vi "crio_FPGA_Antagonist_DMA.vi"() -> ()   [LabVIEW 2019]
uses:
  <vilib>/rvi/Analysis/control/PID/Typedef/niFpgaPID_PIGains.ctl
  <vilib>/rvi/Analysis/control/PID/Typedef/niFpgaPID_ManualControl.ctl
  hx711/Data.ctl
  hx711/State.ctl
  <vilib>/rvi/Analysis/control/PID/Typedef/niFpgaPID_OutputRange.ctl
  <vilib>/rvi/Emulation/niFpgaSctlEmulationGetInTimedLoop.vi
  <vilib>/rvi/Emulation/niFpgaProcessEmulError.vi
  <vilib>/rvi/eio/common/nirviEmuTemplateMethod_errors.vi
  <vilib>/rvi/Emulation/niFpgaGetClockAttributes.vi
  <vilib>/rvi/Emulation/niFpgaEmulationReportErrorSimple.vi
  <vilib>/rvi/Emulation/niFpgaCriticalErrorInLSC.vi
  <vilib>/rvi/Analysis/control/PID/SubVIs/niFpgaPID_PIWrapper.vi
  <vilib>/rvi/interface/RandomDataEmulation/niFpgaRandomDataHandleErrors.vi
  <vilib>/eio/EIOMethodNode/EIOMethodNode.xnode
  <vilib>/eio/EIONode/EIONode.xnode
  <vilib>/rvi/DataTransferAndStorage/Container/XNode/niFpgaContainer.xnode
  <vilib>/rvi/interface/RandomDataEmulation/nirviRandomDataFpgaReadWriteTemplate.vi
panel:
  out "Data array":i32[](array[numeric])
  in  "PowerDown?":bool
  out "Data":i32
  in  "Gain/ChannelSelect":T1(ring)=enum."Channel A/Gain 64"
  in  "Initial Position":i16=1
  out "Platform Position":i16=20000
  in  "Stepper Direction":bool
  in  "Stepper Enable":bool
  in  "Position Control: Desired Positoin":i16=100
  in  "Manual Operation":bool
  out "Controller Enable":bool
  out "Controller Direction":bool
  in  "mSec to initialize a small push away from limit switch":u32=1 caption="mSec when hit limit"
  in  "mSec when hit limit":u32=100 caption="mSec to pause when hit limit"
  in  "Rail soft limit":i16=10000
  out "Limit Switch":bool
  in  "Half Peirod (pulse 40MHz)":u32=10000 caption="Count(Tick) [Interval between step]"
  out "VCA ControllerPWM Output":sgl
  in  "manual control":T2 {"manual input (0)" scale=-1.0..1.0}
  in  "VCA Position Setpoint":i32
  in  "gains":T3 {"proportional gain" step=0.125}
  in  "Loop Timer DAQ 2":u32=1 caption="Loop Time(uSec)"
  in  "VCA Position Reset":bool
  out "Position (Counts) VCA":i64
  out "B VCA":bool
  out "A VCA":bool
  out "B' VCA":bool
  out "A' VCA":bool
  in  "Velocity Interval (uSec)":u32=1000
  out "Acceleration (Counts/Interval) VCA":i32
  out "Velocity (Counts/Interval) VCA":i32
  in  "DC PWM Period (microsec)":i16=50
  in  "LAC Position":u32(slide)=828 scale=1000.0..2000.0
  in  "Count(uSec)":u32=2000
  in  "stop":bool
  in  "Debug: ConnectorA/DIO15":bool
  in  "Debug: ConnectorA/DIO14":bool
  in  "Encoder Debug":bool
  in  "Loop Timer DAQ":u32=1 caption="Loop Time(uSec)"
  in  "LAC Position Reset":bool
  out "Position (Counts)":i64
  out "B":bool
  out "A":bool
  out "B'":bool
  out "A'":bool
  in  "Velocity Interval (uSec)":u32=1000
  out "Acceleration (Counts/Interval)":i32
  out "Velocity (Counts/Interval)":i32
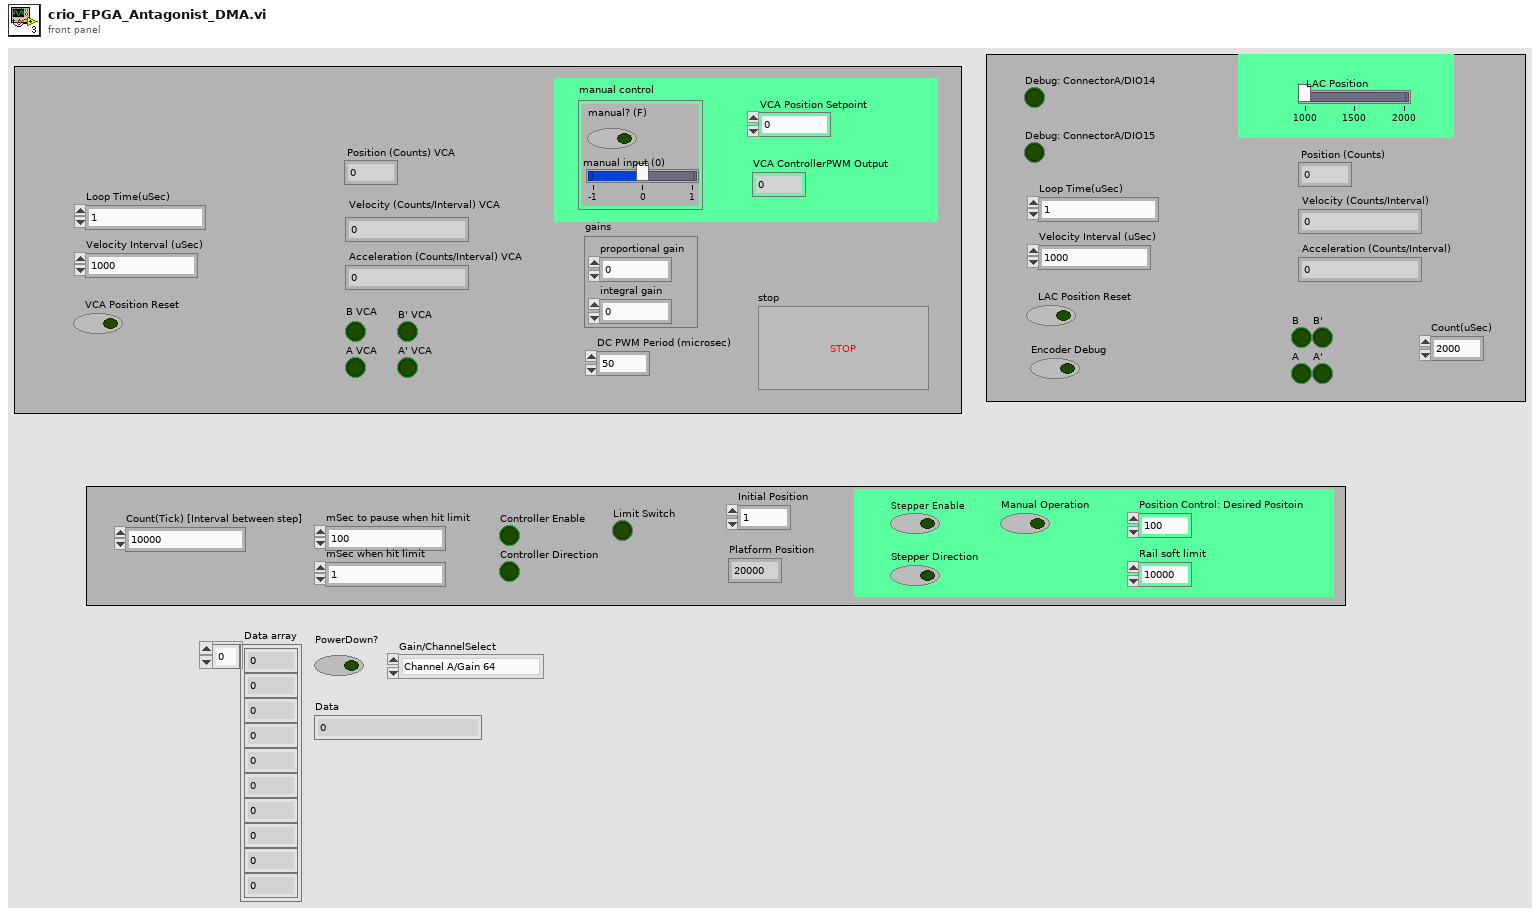
[diagram p1: front panel]
types:
  T1 = enum16{"Channel A/Gain 128", "Channel A/Gain 64", "Channel B/Gain 32"}
  T2 = typedef "niFpgaPID_ManualControl.ctl" = cluster{"manual? (F)":bool, "manual input (0)":sgl}
  T3 = typedef "niFpgaPID_PIGains.ctl" = cluster{"proportional gain":sgl, "integral gain":sgl}
  T4 = typedef "State.ctl" = enum16{"PowerUp", "PowerDown", "Gain/ChannelSelect", "ReadData", "ClockLow", "ClockHigh", "ConvertData", "RetrievalReady?"}
  T5 = typedef "Data.ctl" = cluster{"DT":bool, "SCK":bool, "2's Data":i32, "PulseCount":u8, "DelayTime":u8, "Data":i32, "PowerDown?":bool, "Gain/ChannelSelect":enum16{"Channel A/Gain 128", "Channel A/Gain 64", "Channel B/Gain 32"}}
  T6 = typedef "niFpgaPID_OutputRange.ctl" = cluster{"output high (Inf)":sgl, "output low (-Inf)":sgl}
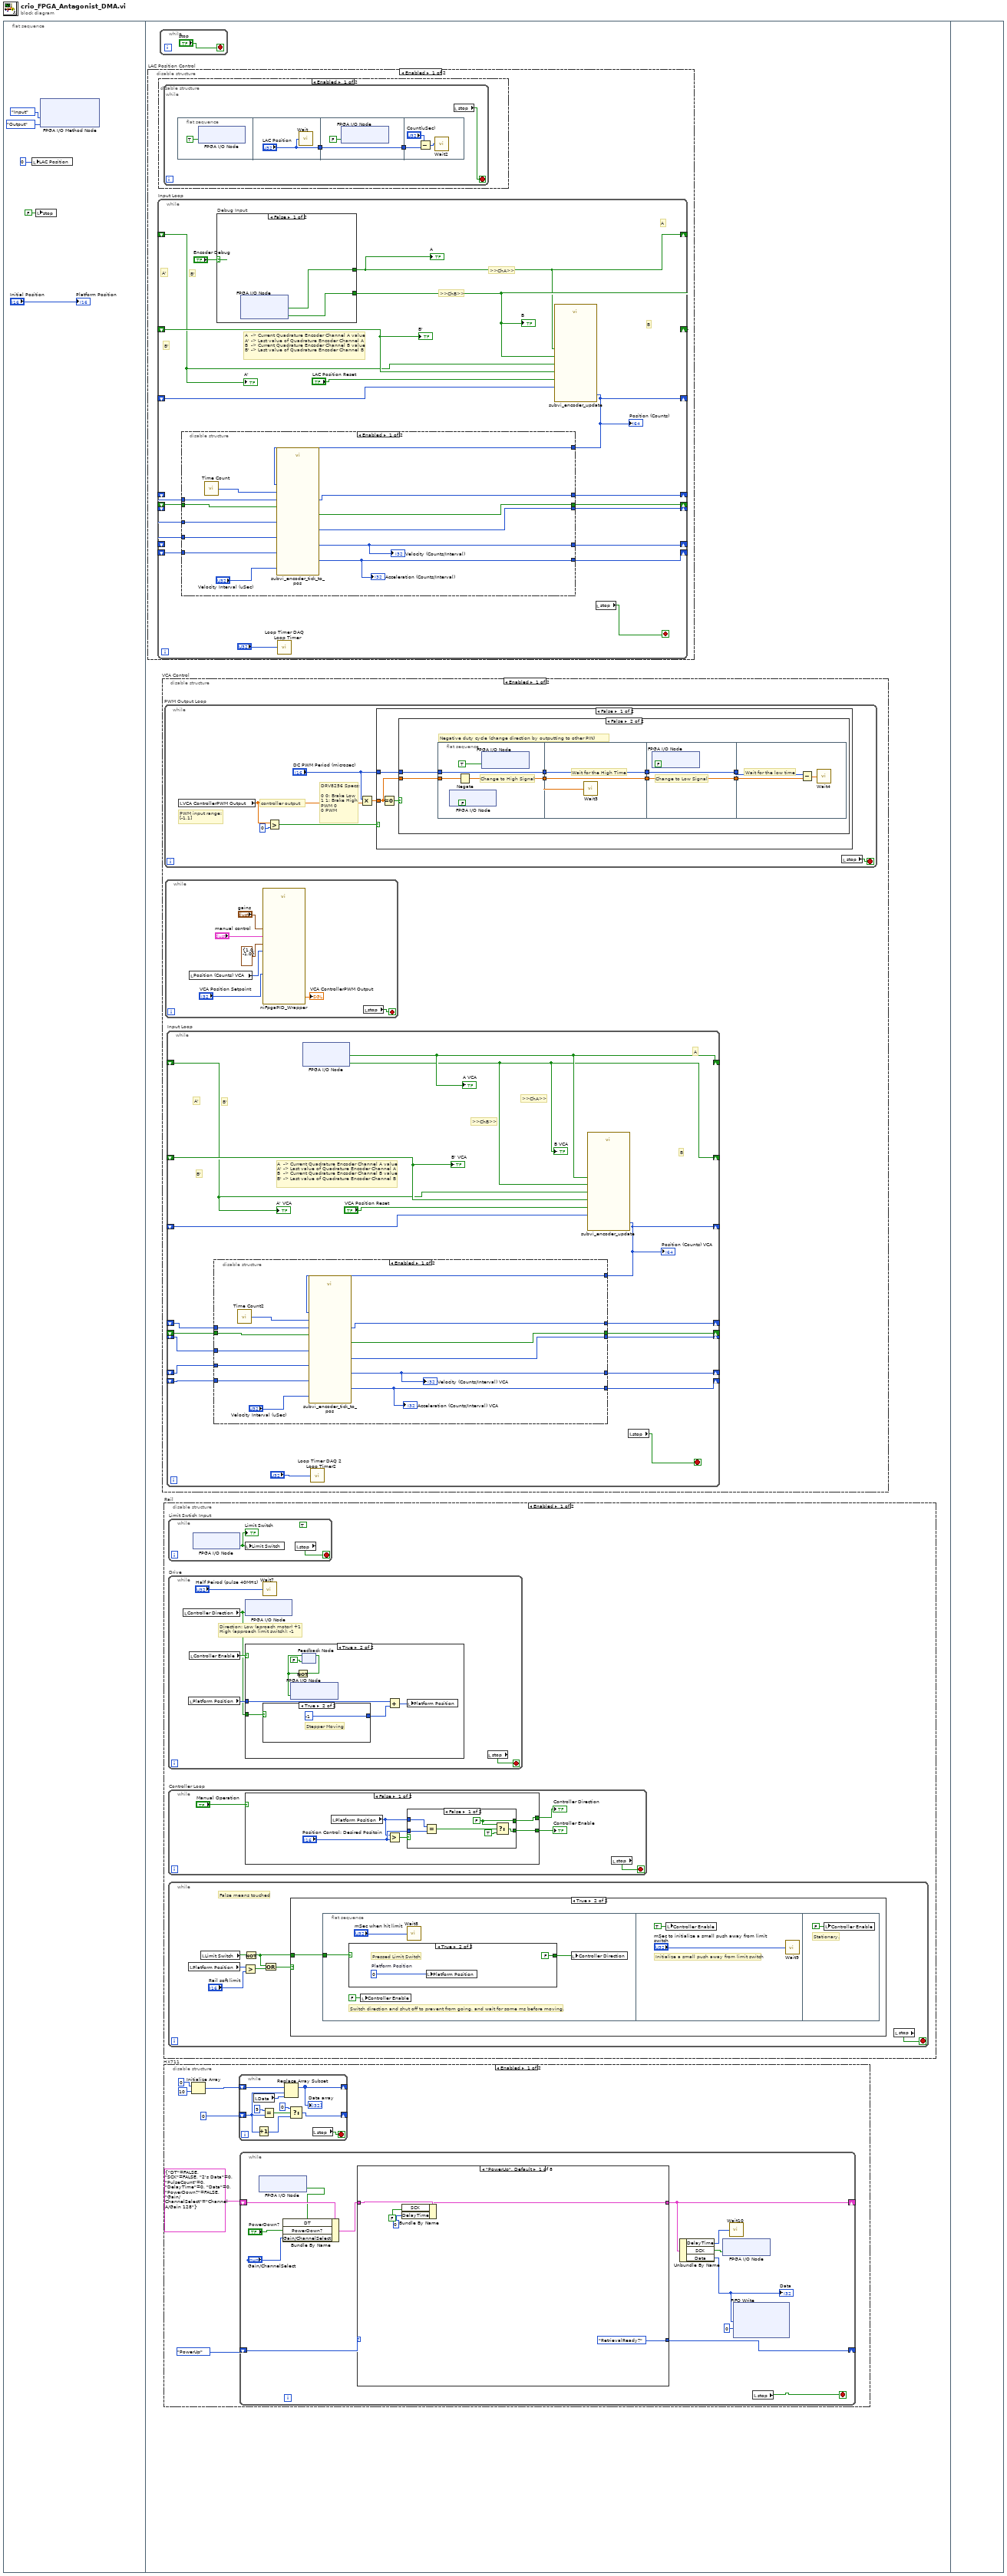
[diagram p0: block diagram]
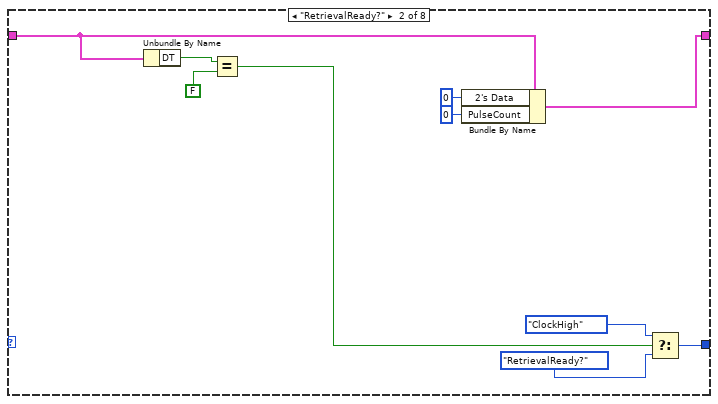
[diagram p2: hidden frame]
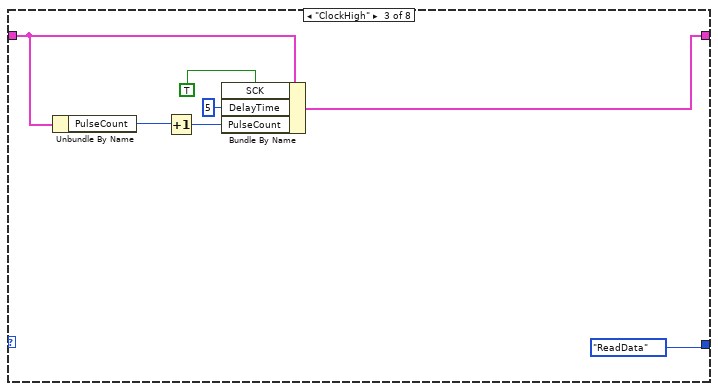
[diagram p3: hidden frame]
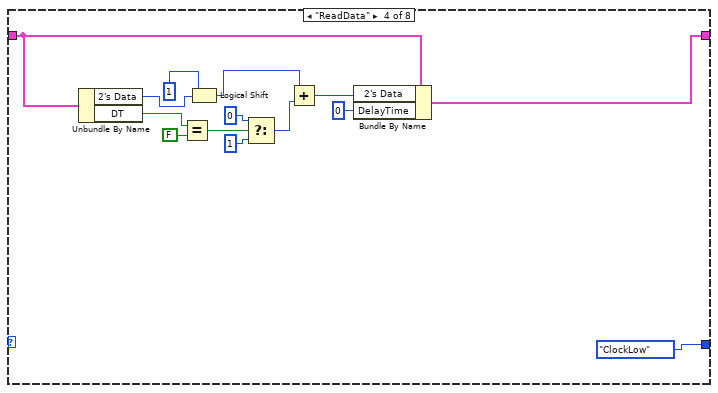
[diagram p4: hidden frame]
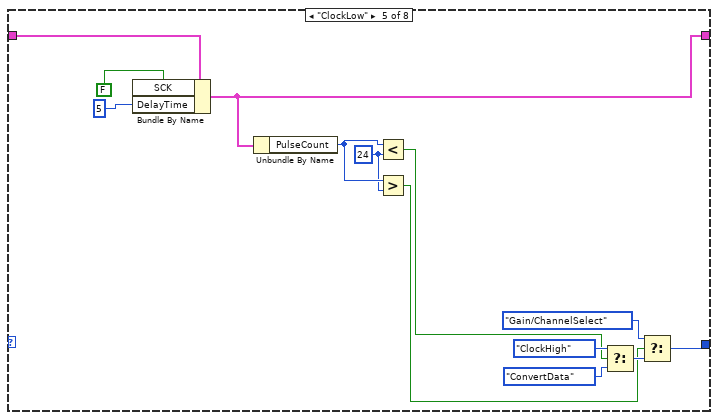
[diagram p5: hidden frame]
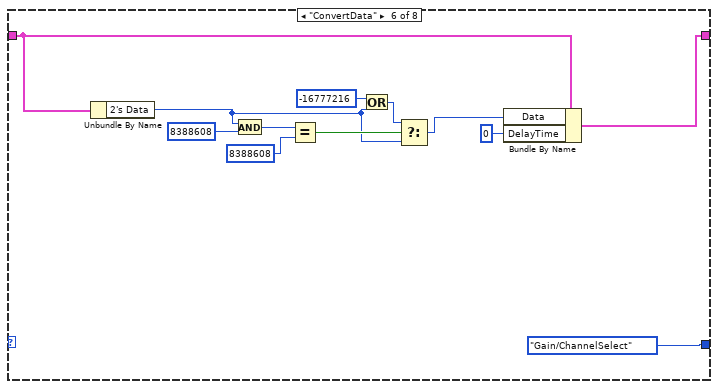
[diagram p6: hidden frame]
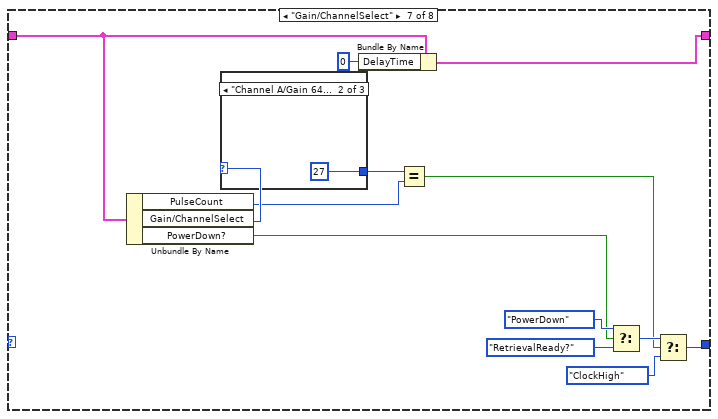
[diagram p7: hidden frame]
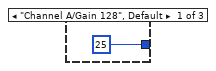
[diagram p8: hidden frame]
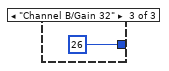
[diagram p9: hidden frame]
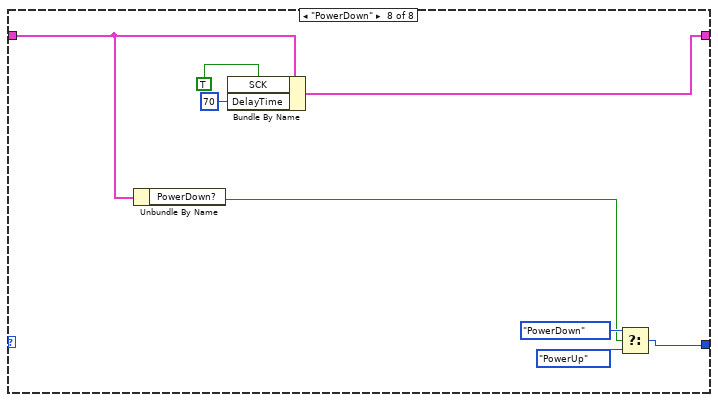
[diagram p10: hidden frame]
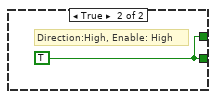
[diagram p12: hidden frame]
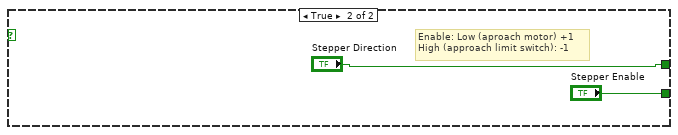
[diagram p13: hidden frame]
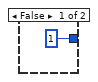
[diagram p15: hidden frame]
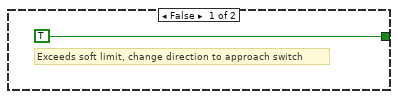
[diagram p17: hidden frame]
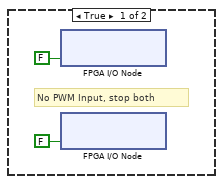
[diagram p20: hidden frame]
diagram:
  n1 = flat-sequence {
    frame #0 {
      n2 = local write "LAC Position"(u32 0 ("Servo wait time")) -> ()
      n3 = local write "stop"(FALSE ("stop")) -> ()
      n4 = xnode "FPGA I/O Method Node"("DIO 7:4"=enum8{"No Change", "Input", "Output"}."Input", "DIO 3:0"=enum8{"No Change", "Input", "Output"}."Output") -> ()  [unwired: 1 in, 1 out]
      "Platform Position" <- "Initial Position"
    }
    frame #1 {
      n5 = disable-structure "LAC Position Control" shown="Enabled" {
        frame Enabled {
          n6 = while "Input Loop" {
            shift-right: [w287] -> _
            shift-left: _ -> [w290]
            shift-right: [w286] -> _
            shift-left: _ -> [w289]
            shift-right: [w282] -> _
            shift-left: _ -> [w288]
            shift-right: [w275] -> _
            shift-left: _ -> [w285]
            shift-right: [w276] -> _
            shift-left: _ -> [w284]
            shift-right: [w283] -> _
            shift-left: _ -> [w281]
            shift-right: [w280] -> _
            shift-left: _ -> [w279]
            shift-right: [w278] -> _
            shift-left: _ -> [w277]
            stop <- w274 stop-if-true
            # "B'"
            # ">>ChB>>"
            # ">>ChA>>"
            # "A'"
            # "A  -> Current Quadrature Encoder Channel A value\nA' -> Last value of Quadrature Encoder Channel A\nB  -> Current Quadrature Encoder Channel B value\nB' -> Last value of Quadrature Encoder Channel B"
            # "B'"
            # "B"
            # "A"
            n7 = case "Debug Input" shown="False" "Encoder Debug" {
              tunnel: [w308 "Debug: ConnectorA/DIO15"] -> w286
              tunnel: [w307 "Debug: ConnectorA/DIO14"] -> w287
              frame False {
                n8 = xnode "FPGA I/O Node"() -> ("Mod1/DIO6"=w308:bool, "Mod1/DIO7"=w307:bool)  [unwired: 2 in, 2 out]
              }
              frame True {
              }
            }
            "B" <- w287
            "A" <- w286
            n9 = call "Loop Timer"("Count(uSec)"="Loop Timer DAQ") -> ()  [unwired: 1 out]
            n10 = call "subvi_encoder_update.vi"("Position Reset"="LAC Position Reset", "Tick'"=w288, "A"=w286, "B'"=w290, "A'"=w289, "B"=w287) -> ("Tick"=w282:i32)  [unwired: 5 in]
            "Position (Counts)" <- w282
            n11 = disable-structure shown="Enabled" {
              disable-tunnel: w285 -> [w305 _]
              disable-tunnel: w284 -> [w304 _]
              disable-tunnel: [w303 _] -> w283
              disable-tunnel: w282 -> [w302 _]
              disable-tunnel: w281 -> [w301 _]
              disable-tunnel: [w300 _] -> w280
              disable-tunnel: w279 -> [w299 _]
              disable-tunnel: [w298 _] -> w278
              disable-tunnel: w277 -> [w297 _]
              disable-tunnel: [w295 _] -> w276
              disable-tunnel: [w294 _] -> w275
              frame Enabled {
                n12 = call "Time Count"() -> ("Tick Count(uSec)"=w296:u32)
                n13 = call "subvi_encoder_tick_to_pos.vi"("Velocity Interval (uSec)"="Velocity Interval (uSec)", "Raw Tick"=w302, "Waited?'"=w299, "Tick Count(uSec)'"=w297, "p'"=w301, "Time Count"=w296, "a'"=w304, "v'"=w305) -> ("Waited?"=w300:bool, "Tick Count(uSec)"=w298:u32, "p"=w303:i32, "a"=w295:i32, "v"=w294:i32)  [unwired: 3 in]
                "Acceleration (Counts/Interval)" <- w295
                "Velocity (Counts/Interval)" <- w294
              }
              frame Disabled {
              }
            }
            n14 = local read "stop"() -> (w274:bool)
            "B'" <- w290
            "A'" <- w289
          }
          n15 = disable-structure shown="Enabled" {
            frame Enabled {
              n16 = while {
                stop <- w264 stop-if-true
                n17 = flat-sequence {
                  tunnel: ["LAC Position"] -> w265
                  tunnel: [w269] -> w266
                  tunnel: w265 -> [w269]
                  tunnel: w266 -> [w273]
                  frame #0 {
                    n18 = xnode "FPGA I/O Node"("Mod8/DIO5"=TRUE) -> ()  [unwired: 1 in, 1 out]
                  }
                  frame #1 {
                    n19 = call "Wait"("Count(uSec)"="LAC Position") -> ()  [unwired: 1 out]
                  }
                  frame #2 {
                    n20 = xnode "FPGA I/O Node"("Mod8/DIO5"=FALSE) -> ()  [unwired: 1 in, 1 out]
                  }
                  frame #3 {
                    n21 = Subtract(x="Count(uSec)", y=w273) -> (x-y=w272:u32)
                    n22 = call "Wait2"("Count(uSec)"=w272) -> ()  [unwired: 1 out]
                  }
                }
                n23 = local read "stop"() -> (w264:bool)
              }
            }
            frame Disabled {
            }
          }
        }
        frame Disabled {
        }
      }
      n24 = while {
        stop <- "stop" stop-if-true
      }
      n25 = disable-structure "VCA Control" shown="Enabled" {
        frame Enabled {
          n26 = while "PWM Output Loop" {
            stop <- w212 stop-if-true
            # "PWM input range:\n[-1,1]"
            # "DRV8256 Specs:\n\n0 0: Brake Low\n1 1: Brake High\nPWM 0\n0 PWM"
            # "controller output"
            n27 = local read "VCA ControllerPWM Output"() -> (w213:sgl)
            n28 = Greater?(x=w213, y=i16 0) -> (0:w216:bool)
            n29 = Multiply(x="DC PWM Period (microsec)", y=w213) -> (x*y=w215:sgl)
            n30 = case shown="False" w216 {
              tunnel: w215 -> [w220 w251]
              tunnel: "DC PWM Period (microsec)" -> [w218 w250]
              frame False {
                n31 = Equal To 0?(x=w220) -> (x = 0?=w219:bool)
                n32 = case shown="False" w219 {
                  tunnel: w220 -> [_ w230]
                  tunnel: w218 -> [_ w223]
                  frame True {
                    # "No PWM Input, stop both"
                    n33 = xnode "FPGA I/O Node"("Mod1/DIO1"=FALSE) -> ()  [unwired: 1 in, 1 out]
                    n34 = xnode "FPGA I/O Node"("Mod1/DIO0"=FALSE) -> ()  [unwired: 1 in, 1 out]
                  }
                  frame False {
                    # "Negative duty cycle (change direction by outputting to other PIN)"
                    n35 = flat-sequence {
                      tunnel: w230 -> [w233]
                      tunnel: [w232] -> w229
                      tunnel: [w231] -> w224
                      tunnel: w223 -> [w231]
                      tunnel: w229 -> [w237]
                      tunnel: [w237] -> w228
                      tunnel: [w236] -> w225
                      tunnel: w224 -> [w236]
                      tunnel: w228 -> [w239]
                      tunnel: [w239] -> w227
                      tunnel: [w238] -> w226
                      tunnel: w225 -> [w238]
                      tunnel: w227 -> [w243]
                      tunnel: w226 -> [w242]
                      frame #0 {
                        # "Change to High Signal"
                        n36 = xnode "FPGA I/O Node"("Mod1/DIO0"=FALSE) -> ()  [unwired: 1 in, 1 out]
                        n37 = Negate(x=w233) -> (-x=w232:sgl)
                        n38 = xnode "FPGA I/O Node"("Mod1/DIO1"=TRUE) -> ()  [unwired: 1 in, 1 out]
                      }
                      frame #1 {
                        # "Wait for the High Time"
                        n39 = call "Wait3"("Count(uSec)"=w237) -> ()  [unwired: 1 out]
                      }
                      frame #2 {
                        # "Change to Low Signal"
                        n40 = xnode "FPGA I/O Node"("Mod1/DIO1"=FALSE) -> ()  [unwired: 1 in, 1 out]
                      }
                      frame #3 {
                        # "Wait for the low time"
                        n41 = Subtract(x=w242, y=w243) -> (x-y=w241:sgl)
                        n42 = call "Wait4"("Count(uSec)"=w241) -> ()  [unwired: 1 out]
                      }
                    }
                  }
                }
              }
              frame True {
                n43 = flat-sequence {
                  tunnel: w251 -> [w252]
                  tunnel: w250 -> [w253]
                  tunnel: [w253] -> w247
                  tunnel: [w252] -> w246
                  tunnel: [w257] -> w248
                  tunnel: w247 -> [w257]
                  tunnel: w246 -> [w256]
                  tunnel: [w256] -> w245
                  tunnel: [w259] -> w249
                  tunnel: w248 -> [w259]
                  tunnel: w245 -> [w258]
                  tunnel: [w258] -> w244
                  tunnel: w249 -> [w263]
                  tunnel: w244 -> [w261]
                  frame #0 {
                    # "Change to High Signal"
                    n44 = xnode "FPGA I/O Node"("Mod1/DIO1"=FALSE ("ConnectorB/DIO9")) -> ()  [unwired: 1 in, 1 out]
                    n45 = xnode "FPGA I/O Node"("Mod1/DIO0"=TRUE) -> ()  [unwired: 1 in, 1 out]
                  }
                  frame #1 {
                    # "Wait for the high time"
                    n46 = call "Wait5"("Count(uSec)"=w256) -> ()  [unwired: 1 out]
                  }
                  frame #2 {
                    # "Turn off"
                    n47 = xnode "FPGA I/O Node"("Mod1/DIO0"=FALSE) -> ()  [unwired: 1 in, 1 out]
                  }
                  frame #3 {
                    # "Wait for the low time"
                    n48 = Subtract(x=w263, y=w261) -> (x-y=w262:sgl)
                    n49 = call "Wait6"("Count(uSec)"=w262) -> ()  [unwired: 1 out]
                  }
                }
              }
            }
            n50 = local read "stop"() -> (w212:bool)
          }
          n51 = while {
            stop <- w211 stop-if-true
            n52 = local read "Position (Counts) VCA"() -> (w210:i64)
            n53 = call-poly <vilib>:"niFpgaPID_Wrapper.vi"("setpoint"="VCA Position Setpoint", "process variable"=w210, "manual control"="manual control", "gains"="gains", "output range"=T6 {"output high (Inf)"=1.0, "output low (-Inf)"=-1.0}) -> ("output"=→"VCA ControllerPWM Output":sgl)  [unwired: 8 in, 2 out]
            n54 = local read "stop"() -> (w211:bool)
          }
          n55 = while "Input Loop" {
            shift-right: [w173] -> _
            shift-left: _ -> [w189]
            shift-right: [w174] -> _
            shift-left: _ -> [w188]
            shift-right: [w183] -> _
            shift-left: _ -> [w187]
            shift-right: [w176] -> _
            shift-left: _ -> [w186]
            shift-right: [w177] -> _
            shift-left: _ -> [w185]
            shift-right: [w184] -> _
            shift-left: _ -> [w182]
            shift-right: [w181] -> _
            shift-left: _ -> [w180]
            shift-right: [w179] -> _
            shift-left: _ -> [w178]
            stop <- w175 stop-if-true
            # "B'"
            # ">>ChB>>"
            # ">>ChA>>"
            # "A'"
            # "A  -> Current Quadrature Encoder Channel A value\nA' -> Last value of Quadrature Encoder Channel A\nB  -> Current Quadrature Encoder Channel B value\nB' -> Last value of Quadrature Encoder Channel B"
            # "B'"
            # "B"
            # "A"
            n56 = xnode "FPGA I/O Node"() -> ("Mod1/DIO4"=w174:bool, "Mod1/DIO5"=w173:bool)  [unwired: 2 in, 2 out]
            "B VCA" <- w173
            "A VCA" <- w174
            n57 = call "Loop Timer2"("Count(uSec)"="Loop Timer DAQ 2") -> ()  [unwired: 1 out]
            n58 = call "subvi_encoder_update.vi"("Position Reset"="VCA Position Reset", "Tick'"=w187, "A"=w174, "B'"=w189, "A'"=w188, "B"=w173) -> ("Tick"=w183:i32)  [unwired: 5 in]
            "Position (Counts) VCA" <- w183
            n59 = disable-structure shown="Enabled" {
              disable-tunnel: w186 -> [w203 _]
              disable-tunnel: w185 -> [w202 _]
              disable-tunnel: [w201 _] -> w184
              disable-tunnel: w183 -> [w200 _]
              disable-tunnel: w182 -> [w199 _]
              disable-tunnel: [w198 _] -> w181
              disable-tunnel: w180 -> [w197 _]
              disable-tunnel: [w196 _] -> w179
              disable-tunnel: w178 -> [w195 _]
              disable-tunnel: [w193 _] -> w177
              disable-tunnel: [w192 _] -> w176
              frame Enabled {
                n60 = call "Time Count2"() -> ("Tick Count(uSec)"=w194:u32)
                n61 = call "subvi_encoder_tick_to_pos.vi"("Velocity Interval (uSec)"="Velocity Interval (uSec)", "Raw Tick"=w200, "Waited?'"=w197, "Tick Count(uSec)'"=w195, "p'"=w199, "Time Count"=w194, "a'"=w202, "v'"=w203) -> ("Waited?"=w198:bool, "Tick Count(uSec)"=w196:u32, "p"=w201:i32, "a"=w193:i32, "v"=w192:i32)  [unwired: 3 in]
                "Acceleration (Counts/Interval) VCA" <- w193
                "Velocity (Counts/Interval) VCA" <- w192
              }
              frame Disabled {
              }
            }
            n62 = local read "stop"() -> (w175:bool)
            "B' VCA" <- w189
            "A' VCA" <- w188
          }
        }
        frame Disabled {
        }
      }
      n63 = disable-structure "Rail" shown="Enabled" {
        frame Enabled {
          n64 = while "Limit Swtich Input" {
            stop <- w171 stop-if-true
            (unwired) TRUE ("Mod8/DIO2")
            n65 = xnode "FPGA I/O Node"() -> ("Mod8/DIO2"=w172:bool)  [unwired: 1 in, 1 out]
            "Limit Switch" <- w172
            n66 = local write "Limit Switch"(w172) -> ()
            n67 = local read "stop"() -> (w171:bool)
          }
          n68 = while "Drive" {
            stop <- w139 stop-if-true
            # "Direction: Low (aproach motor) +1\nHigh (approach limit switch): -1"
            n69 = local read "Controller Direction"() -> (w140:bool)
            n70 = local read "Platform Position"() -> (w142:i16)
            n71 = local read "Controller Enable"() -> (w141:bool)
            n72 = xnode "FPGA I/O Node"("Mod8/DIO4"=w140) -> ()  [unwired: 1 in, 1 out]
            n73 = case shown="True" w141 {
              tunnel: w140 -> [_ w147]
              tunnel: w142 -> [_ w144]
              frame False {
              }
              frame True {
                n74 = case shown="True" w147 {
                  tunnel: [i16 1 i16 -1] -> w146
                  frame False {
                  }
                  frame True {
                    # "Stepper Moving"
                  }
                }
                n75 = feedback #1(FALSE ("Connector0/DIO0")) -> (w148:bool)
                n76 = xnode "FPGA I/O Node"("Mod8/DIO3"=w148) -> ()  [unwired: 1 in, 1 out]
                n77 = Not(x=w148) -> (.not. x?=w149:bool)
                n78 = feedback-in #1(w149) -> ()
                n79 = Add(x=w144, y=w146) -> (x+y=w145:i16)
                n80 = local write "Platform Position"(w145) -> ()
              }
            }
            n81 = call "Wait7"("Count(Ticks)"="Half Peirod (pulse 40MHz)") -> ()  [unwired: 1 out]
            n82 = local read "stop"() -> (w139:bool)
          }
          n83 = while "Controller Loop" {
            stop <- w124 stop-if-true
            n84 = case shown="False" "Manual Operation" {
              tunnel: [w128 "Stepper Enable"] -> w122
              tunnel: [w127 "Stepper Direction"] -> w121
              frame False {
                n85 = local read "Platform Position"() -> (w125:i16)
                n86 = Greater?(x=w125, y="Position Control: Desired Positoin") -> (0:w129:bool)
                n87 = case shown="False" w129 {
                  tunnel: [w132 w136] -> w128
                  tunnel: [w130 w136] -> w127
                  tunnel: "Position Control: Desired Positoin" -> [w135 _]
                  tunnel: w125 -> [w134 _]
                  frame False {
                    w130 = FALSE
                    n88 = Equal?(x=w134, y=w135) -> (x = y?=w133:bool)
                    n89 = Select(t=w130, s=w133, f=TRUE) -> (s? t:f=w132:bool)
                  }
                  frame True {
                    w136 = TRUE
                    # "Direction:High, Enable: High"
                  }
                }
              }
              frame True {
                # "Enable: Low (aproach motor) +1\nHigh (approach limit switch): -1"
              }
            }
            "Controller Enable" <- w122
            "Controller Direction" <- w121
            n90 = local read "stop"() -> (w124:bool)
          }
          n91 = while {
            stop <- w159 stop-if-true
            # "False means touched"
            n92 = local read "Platform Position"() -> (w158:i16)
            n93 = local read "Limit Switch"() -> (w154:bool)
            n94 = Greater?(x=w158, y="Rail soft limit") -> (0:w156:bool)
            n95 = Not(x=w154) -> (.not. x?=w153:bool)
            n96 = Or(x=w153, y=w156) -> (x .or. y?=w155:bool)
            n97 = case shown="True" w155 {
              tunnel: w153 -> [_ w160]
              frame False {
                # "Do nothing"
              }
              frame True {
                n98 = flat-sequence {
                  tunnel: w160 -> [w161]
                  frame #0 {
                    # "Switch direction and shut off to prevent from going, and wait for some ms before moving."
                    n99 = case shown="True" w161 {
                      tunnel: [TRUE ("Stepper Direction") FALSE ("Stepper Direction")] -> w162
                      frame False {
                        # "Exceeds soft limit, change direction to approach switch"
                      }
                      frame True {
                        w167 = i16 0  # Platform Position
                        # "Pressed Limit Switch"
                        n100 = local write "Platform Position"(w167) -> ()
                      }
                    }
                    n101 = local write "Controller Enable"(FALSE ("Stepper Direction")) -> ()
                    n102 = call "Wait8"("Count(mSec)"="mSec when hit limit") -> ()  [unwired: 1 out]
                    n103 = local write "Controller Direction"(w162) -> ()
                  }
                  frame #1 {
                    # "Initialize a small push away from limit switch"
                    n104 = local write "Controller Enable"(TRUE ("Stepper Enable")) -> ()
                    n105 = call "Wait9"("Count(mSec)"="mSec to initialize a small push away from limit switch") -> ()  [unwired: 1 out]
                  }
                  frame #2 {
                    # "Stationary."
                    n106 = local write "Controller Enable"(FALSE ("Stepper Enable")) -> ()
                  }
                }
              }
            }
            n107 = local read "stop"() -> (w159:bool)
          }
        }
        frame Disabled {
        }
      }
      n108 = disable-structure "HX711" shown="Enabled" {
        frame Enabled {
          n109 = Initialize Array(0 ("Data"), 10 ("dimension size")) -> (w12:i32[])
          n110 = while {
            shift-right: [w112] -> _
            shift-left: w12 -> [w113]
            shift-right: [w118] -> _
            shift-left: 0 ("index") -> [w114]
            stop <- w111 stop-if-true
            n111 = local read "Data"() -> (w120:i32)
            n112 = Increment(x=w114) -> (x+1=w117:i32)
            n113 = Equal?(x=9, y=w114) -> (x = y?=w115:bool)
            n114 = Replace Array Subset(array=w113, new element=w120, index=w114) -> (w112:i32[])
            "Data array" <- w112
            n115 = Select(t=0 ("index"), s=w115, f=w117) -> (s? t:f=w118:i32)
            n116 = local read "stop"() -> (w111:bool)
          }
          n117 = while {
            shift-right: [w17] -> _
            shift-left: T5 {"DT"=FALSE, "SCK"=FALSE, "2's Data"=0, "PulseCount"=0, "DelayTime"=0, "Data"=0, "PowerDown?"=FALSE, "Gain/ChannelSelect"=enum."Channel A/Gain 128"} ("Data") -> [w22]
            shift-right: [w23] -> _
            shift-left: State."PowerUp" ("State") -> [w25]
            stop <- w15 stop-if-true
            n118 = xnode "FPGA I/O Node"() -> ("Mod8/DIO0"=w20:bool)  [unwired: 1 in, 1 out]
            n119 = Bundle By Name(cluster=w22, "DT"=w20, "PowerDown?"="PowerDown?", "Gain/ChannelSelect"="Gain/ChannelSelect") -> (w21:T5)
            n120 = case shown="\"PowerUp\", Default" w25 {
              tunnel: w21 -> [w30 w34 w43 w48 w74 w79 w89 w104]
              tunnel: [w28 w33 w47 w50 w69 w78 w88 w110] -> w17
              tunnel: [State."RetrievalReady?" ("State") w36 State."ReadData" ("State") State."ClockLow" ("State") w70 State."Gain/ChannelSelect" ("State") w96 w105] -> w23
              frame "PowerUp", Default {
                n121 = Bundle By Name(cluster=w30, "SCK"=FALSE, "DelayTime"=u8 0) -> (w28:T5)
              }
              frame "RetrievalReady?" {
                n122 = Unbundle By Name(w34) -> ("DT"=w40:bool)
                n123 = Equal?(x=w40, y=FALSE) -> (x = y?=w35:bool)
                n124 = Bundle By Name(cluster=w34, "2's Data"=0, "PulseCount"=u8 0) -> (w33:T5)
                n125 = Select(t=State."ClockHigh" ("State"), s=w35, f=State."RetrievalReady?" ("State")) -> (s? t:f=w36:T4)
              }
              frame "ClockHigh" {
                n126 = Unbundle By Name(w43) -> ("PulseCount"=w42:u8)
                n127 = Increment(x=w42) -> (x+1=w41:u8)
                n128 = Bundle By Name(cluster=w43, "SCK"=TRUE, "DelayTime"=u8 5, "PulseCount"=w41) -> (w47:T5)
              }
              frame "ReadData" {
                n129 = Unbundle By Name(w48) -> ("2's Data"=w61:i32, "DT"=w59:bool)
                n130 = Equal?(x=w59, y=FALSE ("SCK")) -> (x = y?=w57:bool)
                n131 = Logical Shift(y=i16 1, x=w61) -> (x << y=w56:i32)
                n132 = Select(t=0 ("DelayTime"), s=w57, f=1 ("DelayTime")) -> (s? t:f=w53:i32)
                n133 = Add(x=w56, y=w53) -> (x+y=w52:i32)
                n134 = Bundle By Name(cluster=w48, "2's Data"=w52, "DelayTime"=u8 0) -> (w50:T5)
              }
              frame "ClockLow" {
                w63 = u8 24 ("y")
                n135 = Bundle By Name(cluster=w74, "SCK"=FALSE, "DelayTime"=u8 5) -> (w69:T5)
                n136 = Unbundle By Name(w69) -> ("PulseCount"=w64:u8)
                n137 = Less?(x=w64, y=w63) -> (x < y?=w66:bool)
                n138 = Greater?(x=w64, y=w63) -> (0:w62:bool)
                n139 = Select(t=State."ClockHigh" ("State"), s=w66, f=State."ConvertData" ("State")) -> (s? t:f=w65:T4)
                n140 = Select(t=State."Gain/ChannelSelect" ("State"), s=w62, f=w65) -> (s? t:f=w70:T4)
              }
              frame "ConvertData" {
                n141 = Unbundle By Name(w79) -> ("2's Data"=w80:i32)
                n142 = And(x=w80, y=8388608) -> (x .and. y?=w85:i32)
                n143 = Equal?(x=w85, y=8388608) -> (x = y?=w83:bool)
                n144 = Or(x=-16777216 ("y"), y=w80) -> (x .or. y?=w81:i32)
                n145 = Select(t=w81, s=w83, f=w80) -> (s? t:f=w76:i32)
                n146 = Bundle By Name(cluster=w79, "Data"=w76, "DelayTime"=u8 0) -> (w78:T5)
              }
              frame "Gain/ChannelSelect" {
                n147 = Unbundle By Name(w89) -> ("PulseCount"=w92:u8, "Gain/ChannelSelect"=w94:T1, "PowerDown?"=w95:bool)
                n148 = case shown="\"Channel A/Gain 64\"" w94 {
                  tunnel: [u8 25 ("PulseCount") u8 27 ("PulseCount") u8 26 ("PulseCount")] -> w93
                  frame "Channel A/Gain 128", Default {
                  }
                  frame "Channel A/Gain 64" {
                  }
                  frame "Channel B/Gain 32" {
                  }
                }
                n149 = Bundle By Name(cluster=w89, "DelayTime"=u8 0) -> (w88:T5)
                n150 = Equal?(x=w93, y=w92) -> (x = y?=w90:bool)
                n151 = Select(t=State."PowerDown" ("State"), s=w95, f=State."RetrievalReady?" ("State")) -> (s? t:f=w91:T4)
                n152 = Select(t=w91, s=w90, f=State."ClockHigh" ("State")) -> (s? t:f=w96:T4)
              }
              frame "PowerDown" {
                n153 = Unbundle By Name(w104) -> ("PowerDown?"=w103:bool)
                n154 = Bundle By Name(cluster=w104, "SCK"=TRUE, "DelayTime"=u8 70) -> (w110:T5)
                n155 = Select(t=State."PowerDown" ("State"), s=w103, f=State."PowerUp" ("State")) -> (s? t:f=w105:T4)
              }
            }
            n156 = Unbundle By Name(w17) -> ("DelayTime"=w24:u8, "SCK"=w16:bool, "Data"=w13:i32)
            "Data" <- w13
            n157 = xnode "FPGA I/O Node"("Mod8/DIO1"=w16) -> ()  [unwired: 1 in, 1 out]
            n158 = call "Wait10"("Count(uSec)"=w24) -> ()  [unwired: 1 out]
            n159 = xnode ("FIFO Write")("Element"=w13, "Timeout"=0) -> ()  [unwired: 1 in, 2 out]
            n160 = local read "stop"() -> (w15:bool)
          }
        }
        frame Disabled {
        }
      }
    }
    frame #2 {
    }
  }
